vi "FGV Map Core.vi"(7 "FGV State":T1, 8 "error in":errorcluster, 10 "Instance Key":string, 11 "Instance In":map{string, variant}(c390)) -> (0 "error out":errorcluster, 1 "Instance Not Found ?":bool, 2 "Instance Overwritten ?":bool, 3 "Instance Out":map{string, variant}(c390), 4 "Was Locked ?":bool)   [LabVIEW 2020, in "FGV Map.lvlib"]
uses:
  FGV Map.lvlib
  Controls/FGV Map Core State.ctl
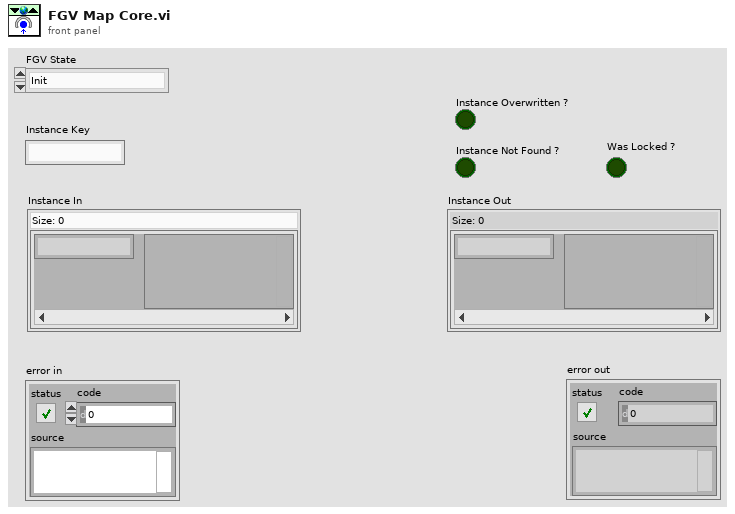
[diagram p1: front panel]
types:
  T1 = typedef "FGV Map.lvlib/FGV Map Core State.ctl" = enum16{"Init", "Set Instance (Unlock)", "Get Instance", "Get Instance (Lock)", "Unlock", "Get All Instances", "Delete Instance"}
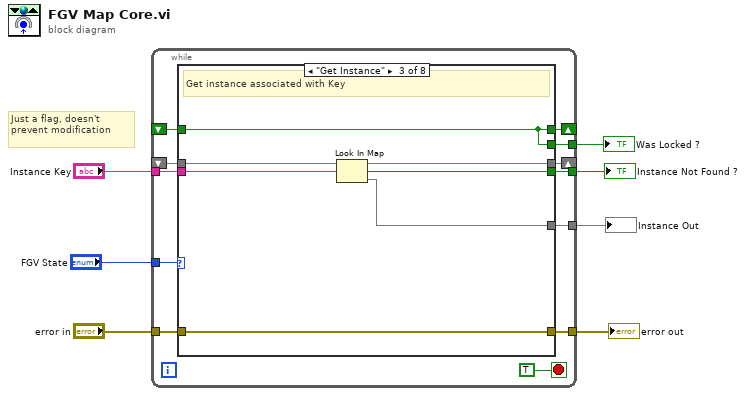
[diagram p0: block diagram]
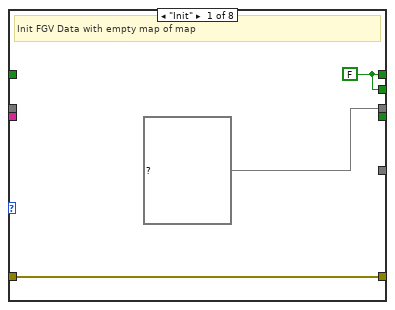
[diagram p2: hidden frame]
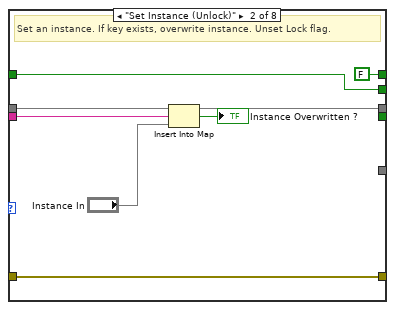
[diagram p3: hidden frame]
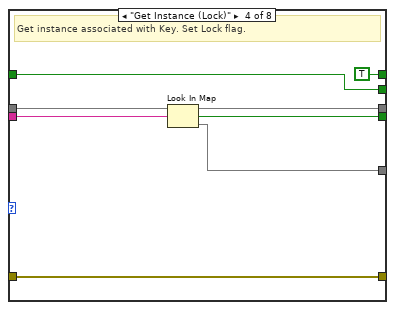
[diagram p4: hidden frame]
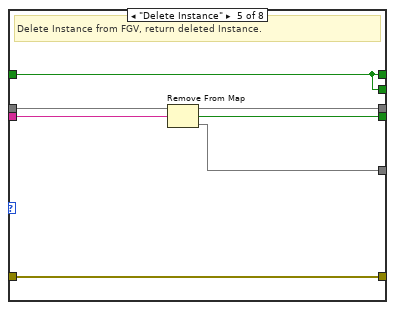
[diagram p5: hidden frame]
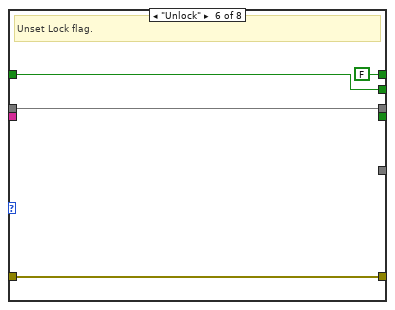
[diagram p6: hidden frame]
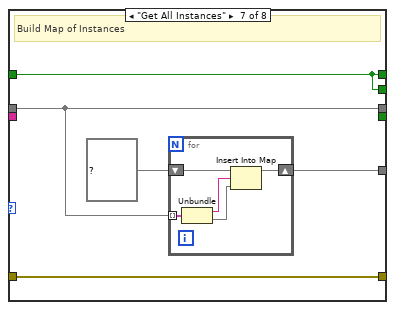
[diagram p7: hidden frame]
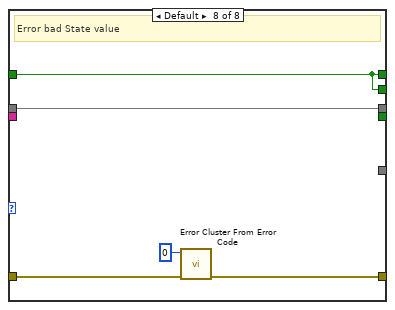
[diagram p8: hidden frame]
diagram:
  # "Just a flag, doesn't prevent modification"
  n1 = while {
    shift-right: [w15] -> _
    shift-left: _ -> [w14]
    tunnel: [w17] -> w7
    tunnel: "error in" -> [w18]
    tunnel: "FGV State" -> [w16]
    tunnel: [w13] -> w4
    tunnel: "Instance Key" -> [w12]
    tunnel: [w11] -> w2
    shift-right: [w10] -> _
    shift-left: _ -> [w9]
    tunnel: [w8] -> w1
    stop <- TRUE stop-if-true
    n2 = case shown="\"Get Instance\"" w16 {
      tunnel: w18 -> [w21 w30 w33 w40 w45 w51 w56 w69]
      tunnel: [w21 w30 w33 w40 w45 w51 w56 w68] -> w17
      tunnel: [map{string, map{string, variant}} {} ("map") w28 w36 w43 w49 w52 w58 w67] -> w15
      tunnel: w14 -> [_ w29 w36 w43 w50 w52 w58 w67]
      tunnel: [_ _ w35 w42 w46 _ w55 _] -> w13
      tunnel: w12 -> [_ w26 w34 w41 w47 _ _ _]
      tunnel: [_ _ w32 w39 w48 _ _ _] -> w11
      tunnel: [w20 FALSE w31 TRUE w44 FALSE w59 w65] -> w10
      tunnel: w9 -> [_ w23 w31 w37 w44 w53 w59 w65]
      tunnel: [w20 w23 w31 w37 w44 w53 w59 w65] -> w8
      frame "Init" {
        w20 = FALSE
        # "Init FGV Data with empty map of map"
      }
      frame "Set Instance (Unlock)" {
        # "Set an instance. If key exists, overwrite instance. Unset Lock flag."
        n3 = Insert Into Map(map in=w29, key=w26, value="Instance In") -> (map out=w28:map{string, map{string, variant}}, key already included?=→"Instance Overwritten ?":bool)  [unwired: 1 out]
      }
      frame "Get Instance" {
        # "Get instance associated with Key"
        n4 = Look In Map(map=w36, key=w34) -> (key not found?=w32:bool, value=w35:map{string, variant})  [unwired: 1 in]
      }
      frame "Get Instance (Lock)" {
        # "Get instance associated with Key. Set Lock flag."
        n5 = Look In Map(map=w43, key=w41) -> (key not found?=w39:bool, value=w42:map{string, variant})  [unwired: 1 in]
      }
      frame "Delete Instance" {
        # "Delete Instance from FGV, return deleted Instance."
        n6 = Remove From Map(10:w47, 11:w50) -> (1:w46:map{string, variant}, 2:w48:bool, 3:w49:map{string, map{string, variant}})
      }
      frame "Unlock" {
        # "Unset Lock flag."
      }
      frame "Get All Instances" {
        # "Build Map of Instances"
        n7 = for {
          tunnel: w58 -> [w62] mode=indexing
          shift-right: [w63] -> w55
          shift-left: map{string, variant} {} ("map") -> [w64]
          n8 = Unbundle(w62) -> ("key"=w60:string, "map"=w61:map{string, variant})
          n9 = Insert Into Map(map in=w64, key=w60, value=w61) -> (map out=w63:map{string, variant})  [unwired: 2 out]
        }
      }
      frame Default {
        # "Error bad State value"
        n10 = call <vilib>:"Error Cluster From Error Code.vi"("error in (no error)"=w69, "error code (0)"=0) -> ("error out"=w68:errorcluster)  [unwired: 7 in]
      }
    }
  }
  "error out" <- w7
  "Instance Out" <- w4
  "Instance Not Found ?" <- w2
  "Was Locked ?" <- w1
